vi "P2.vi"(1 "A2":dbl[](array[numeric]), 2 "A1":dbl[](array[numeric])) -> (0 "A3":dbl[](array[numeric]))   [LabVIEW 2010]
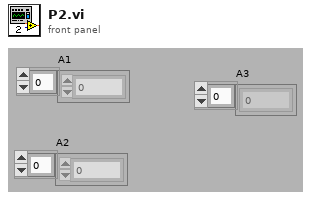
[diagram p1: front panel]
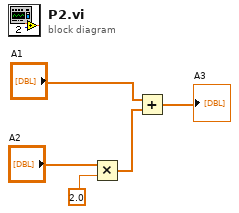
[diagram p0: block diagram]
diagram:
  n1 = Multiply(x="A2", y=2.0) -> (x*y=w2:dbl[])
  n2 = Add(x="A1", y=w2) -> (x+y=→"A3":dbl[])
